vi "COMI DA Set Range.vi"(7 "VMax":i32, 9 "VMin":i32, 10 "ch":i32, 11 "hDevice":u32) -> (3 "hDevice out":u32)   [LabVIEW 2017, in "Comidll.lvlib"]
doc: "void (COMI_DA_SetRange) (HANDLE hDevice, int ch, int VMin, int VMax);"
uses:
  <userlib>/Comidll/Comidll.lvlib
  <userlib>/Comidll/Comidll.dll
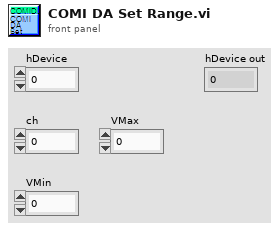
[diagram p1: front panel]
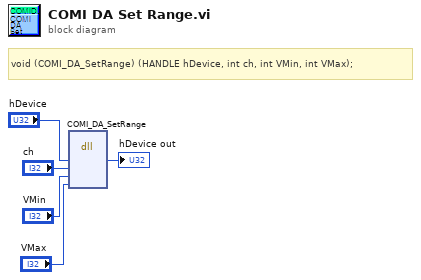
[diagram p0: block diagram]
diagram:
  # "void\t(COMI_DA_SetRange) (HANDLE hDevice, int ch, int VMin, int VMax);"
  n1 = dll-call lib="C:/Program Files/National Instruments/LabVIEW 2017/user.lib/Comidll/Comidll.*" fn="COMI_DA_SetRange"("hDevice"="hDevice", "ch"="ch", "VMin"="VMin", "VMax"="VMax") -> ("hDevice"=→"hDevice out":u32)  [unwired: 7 in, 2 out]
